vi "String EW.vi"(11 "Data In":string) -> (3 "Data Out":string)   [LabVIEW 2016]
uses:
  Core/Assert API Components/Failure Actions.ctl
  Core/Assert API Components/VI References.ctl
  Core/Assert API Components/Assert API Components.lvlib
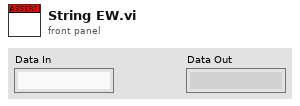
[diagram p1: front panel]
types:
  T1 = typedef "Assert API Components.lvlib/VI References.ctl" = cluster{"Calling VI Ref":refnum<vi>, "Assert VI Ref":refnum<vi>}
  T2 = typedef "Assert API Components.lvlib/Failure Actions.ctl" = enum16{"None", "Log To File", "Pause Execution", "Abort Execution"}
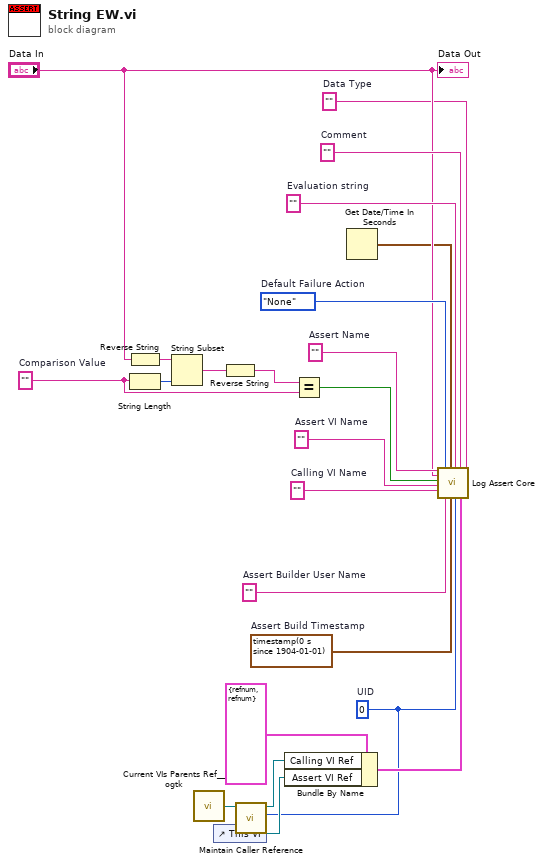
[diagram p0: block diagram]
diagram:
  w1 = 0  # UID
  w4 = ""  # Assert VI Name
  w5 = ""  # Calling VI Name
  w6 = ""  # Data Type
  w7 = ""  # Assert Builder User Name
  w8 = timestamp(0 s since 1904-01-01)  # Assert Build Timestamp
  w21 = ""  # Comment
  w20 = ""  # Evaluation string
  w22 = Failure_Actions."None"  # Default Failure Action
  w23 = ""  # Assert Name
  w16 = ""  # Comparison Value
  n1 = Reverse String(1:"Data In") -> (0:w14:string)
  n2 = String Length(string=w16) -> (length=w18:i32)
  n3 = String Subset(string=w14, length (rest)=w18) -> (substring=w17:string)  [unwired: 1 in]
  n4 = call <userlib>:"Current VIs Parents Ref__ogtk.vi"() -> ("Calling VI's Reference"=w11:refnum<vi>)  [unwired: 2 in]
  n5 = control-ref of="This VI"() -> (w10:refnum<vi>)
  n6 = Reverse String(1:w17) -> (0:w13:string)
  n7 = call "Maintain Caller Reference.vi"("UID"=w1, "VI in"=w11) -> ("VI out"=w2:refnum<vi>)  [unwired: 9 in]
  n8 = Bundle By Name(cluster=T1 {"Calling VI Ref"=refnum, "Assert VI Ref"=refnum} ("VI References"), "Calling VI Ref"=w2, "Assert VI Ref"=w10) -> (w9:T1)
  n9 = Equal?(x=w13, y=w16) -> (x = y?=w15:bool)
  n10 = Get Date/Time In Seconds() -> (seconds since 1Jan1904=w3:timestamp)
  n11 = call "Log Assert Core.vi"("Assert Name"=w23, "Data Value"="Data In", "Status"=w15, "Assert VI Name"=w4, "Calling VI Name"=w5, "Failure Action"=w22, "Assert Builder User Name"=w7, "Last Update"=w3, "Assert Build Timestamp"=w8, "Evaluation String"=w20, "Assert VI UID"=w1, "Comment"=w21, "VI References"=w9, "Data Type"=w6) -> ()  [unwired: 6 in]
  "Data Out" <- "Data In"
